vi "GetColorFilePath.vi"(11 "String":string) -> (0 "name":string, 3 "path":path)   [LabVIEW 2022 SP3]
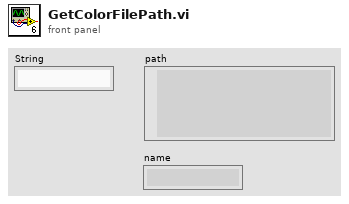
[diagram p1: front panel]
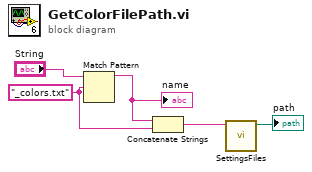
[diagram p0: block diagram]
diagram:
  w3 = "_colors.txt" ("pattern")
  n1 = Match Pattern(string="String", regular expression=w3) -> (before substring=w4:string)  [unwired: 1 in, 3 out]
  "name" <- w4
  n2 = Concatenate Strings(w4, w3) -> (w2:string)
  n3 = call "SettingsFiles.vi"("settings file name"=w2) -> ("file path"=→"path":path)  [unwired: 9 in, 1 out]
